vi "flat.vi"() -> ()   [LabVIEW 2020]
doc: "Recommended Input Signal: 100 kHz, 4 Vpp, sine wave\n\nDevices Supported: Refer to NI Example Finder\n\nThis example configures all the oscilloscope's vertical, horizontal, and triggering properties before every acquisition. It allows you to experiment with numerous configurations, including acquisition types and triggering modes, since it supports nearly the entire functionality of NI-SCOPE. However, it is may be more instructive to consult other examples about specific topics such as FlexRes, Random Interleaved Sampling, and Multi-Record to learn more about these features.\n\nMany parameters are included an the front panel of this example. Notice that the \"min sample rate\" is next to the \"actual sample rate,\" and similarly the \"min record length\" is near the \"actual record length.\" The \"min\" values are specified with the Configure Horizontal Timing VI. NI-SCOPE maintains a constant time per record for each acquisition. So when you specify a min sample rate and a min record length, this determines the amount of time the acquisition should take:\n\n time per record = min record length / min sampling rate. \n\nHowever, oscilloscopes support only a certain number of defined sampling rates, so if the value chosen is not a valid rate, it is rounded to the next higher rate, called the actual sample rate. The actual record length is then calculated in order to maintain the time per record. Both of these values are returned in this example so you can investigate the effects of parameter rounding with your oscilloscope. For more information about parameter coercions, see the NI High Speed Digitizers Help.\n\nThe enforce realtime property allows this example to use Random Interleaved Sampling. See the Random Interleaved Sampling example for more details.\n\nKeep in mind that not all digitizers/oscilloscopes support all the features in this example. The NI High Speed Digitizers Help includes a table of supported features for each device."
uses:
  <instrlib>/niFgen/niFgen.llb/niFgen Output Impedance.ctl
  <instrlib>/niDCPower/nidcpower.llb/niDCPower Source Mode.ctl
  <instrlib>/niDCPower/nidcpower.llb/niDCPower Output Function.ctl
  <instrlib>/niDCPower/nidcpower.llb/niDCPower Wait For Event - Event.ctl
  <instrlib>/niFgen/niFgen.llb/niFgen Output Mode.ctl
  <instrlib>/niFgen/niFgen.llb/niFgen Waveform Type.ctl
  <vilib>/measure/matone.llb/Extract Single Tone Information 1 Chan.vi
  <instrlib>/niScope/Acquire/Fetch/niScope Multi Fetch Cluster.vi
  <vilib>/measure/NI_MAPro.lvlib
panel:
  out "Vout":dbl[](array[numeric])
  out "Vin":dbl[](array[numeric])
  out "CH0 detected frequency":dbl format="%.2p"
  out "CH0 Spectrum(instantaneous)":cluster{"f0":dbl, "df":dbl, dbl[]}(graph)
  in  "Timeout (s)":dbl=5.0 format="%.2f"
  in  "% search":dbl=5.0
  in  "current level range":dbl=0.01 format="%#.6p"
  in  "voltage level range":dbl=10.0 format="%.6p"
  in  "Min record length":i32=1000000
  in  "Min Sample Rate (S/s)":dbl=5000000.0 format="%#_6p"
  in  "Load Current (A)":dbl=-0.01
  in  "Input Voltage (V)":dbl=7.5
  in  "SMU Load":refnum<k15>="SMU_Load"
  in  "SMU Source":refnum<k15>="SMU_Source"
  in  "Max Freq (Hz)":i32=1000000 format="%.0p"
  in  "Min Freq (Hz)":dbl(ring)=100.0 items=["10Hz"=10.0, "100Hz"=100.0, "1kHz"=1000.0, "100kHz"=100000.0]
  out "PSRR vs Frequency Graph":cluster{dbl, dbl}[](graph) caption="Input Voltage :\nLoad current :\nOutput voltage :"
  out "CH0":T1(graph)
  out "PSRR":dbl[](array[numeric])=[nan, nan, nan]
  in  "FGen Vpk-pk (V)":dbl=1.0 format="%#_2f"
  out "Current Freq(Hz)":dbl=300.0
  in  "FGEN Resource Name":refnum<k15>="FGEn"
  in  "Resource Name":refnum<k15>="PXI1Slot5" caption="Scope Resource Name"
  # "LDO_PSRR Measurement"
  # "Debug"
  # "Test Result"
  # "Configuration"
  # "SMU"
  # "Waveform Generator"
  # "Oscilloscope"
  # "Advance"
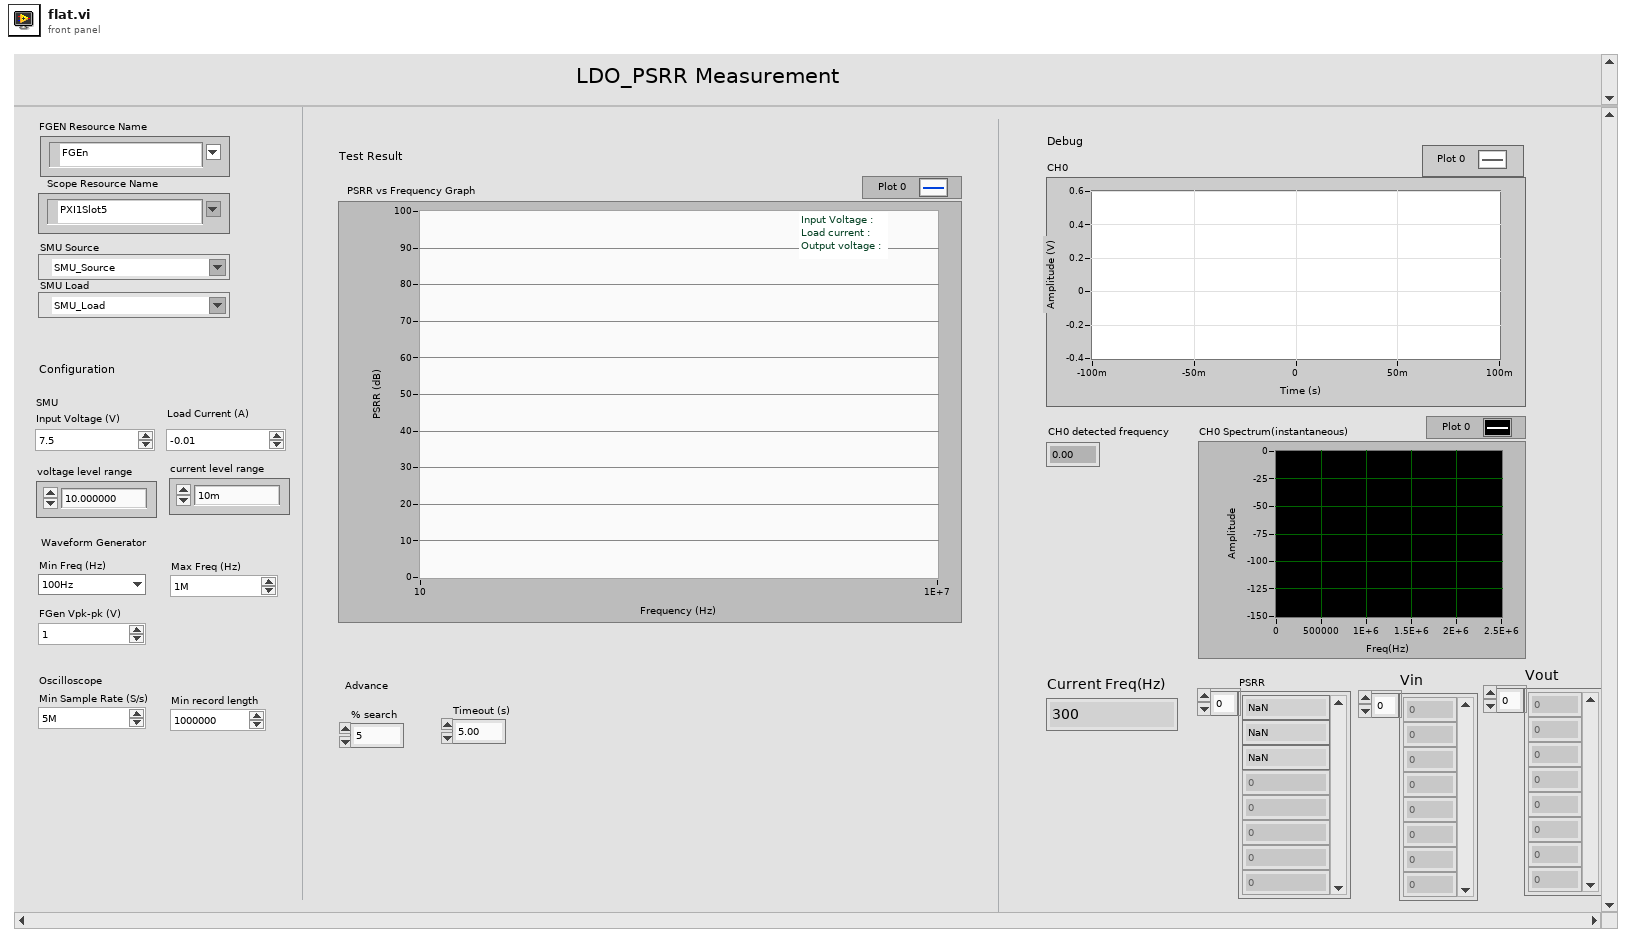
[diagram p1: front panel]
types:
  T1 = cluster{"relativeInitialX":dbl, "xIncrement":dbl, "wfm":dbl[]}
  T2 = typedef "niDCPower Output Function.ctl" = i32
  T3 = typedef "niDCPower Source Mode.ctl" = i32
  T4 = typedef "niDCPower Wait For Event - Event.ctl" = i32
  T5 = typedef "niFgen Output Impedance.ctl" = i32
  T6 = cluster{"approx freq. (optional)":dbl, "search (+/- % of Fsampl.)":dbl}
  T7 = enum32{"none", "input signal", "detected signal", "residual signal"}
  T8 = typedef "niFgen Waveform Type.ctl" = i32
  T9 = typedef "niFgen Output Mode.ctl" = u32
  T10 = cluster{"relativeInitialX":dbl, "xIncrement":dbl, "wfm":dbl[]}[]
  T11 = cluster{"exported time signal":waveform(dbl), "exported spectrum (dB)":cluster{"f0":dbl, "df":dbl, "dB Spectrum (Hann)":dbl[]}}
  T12 = cluster{"f0":dbl, "df":dbl, "dB Spectrum (Hann)":dbl[]}
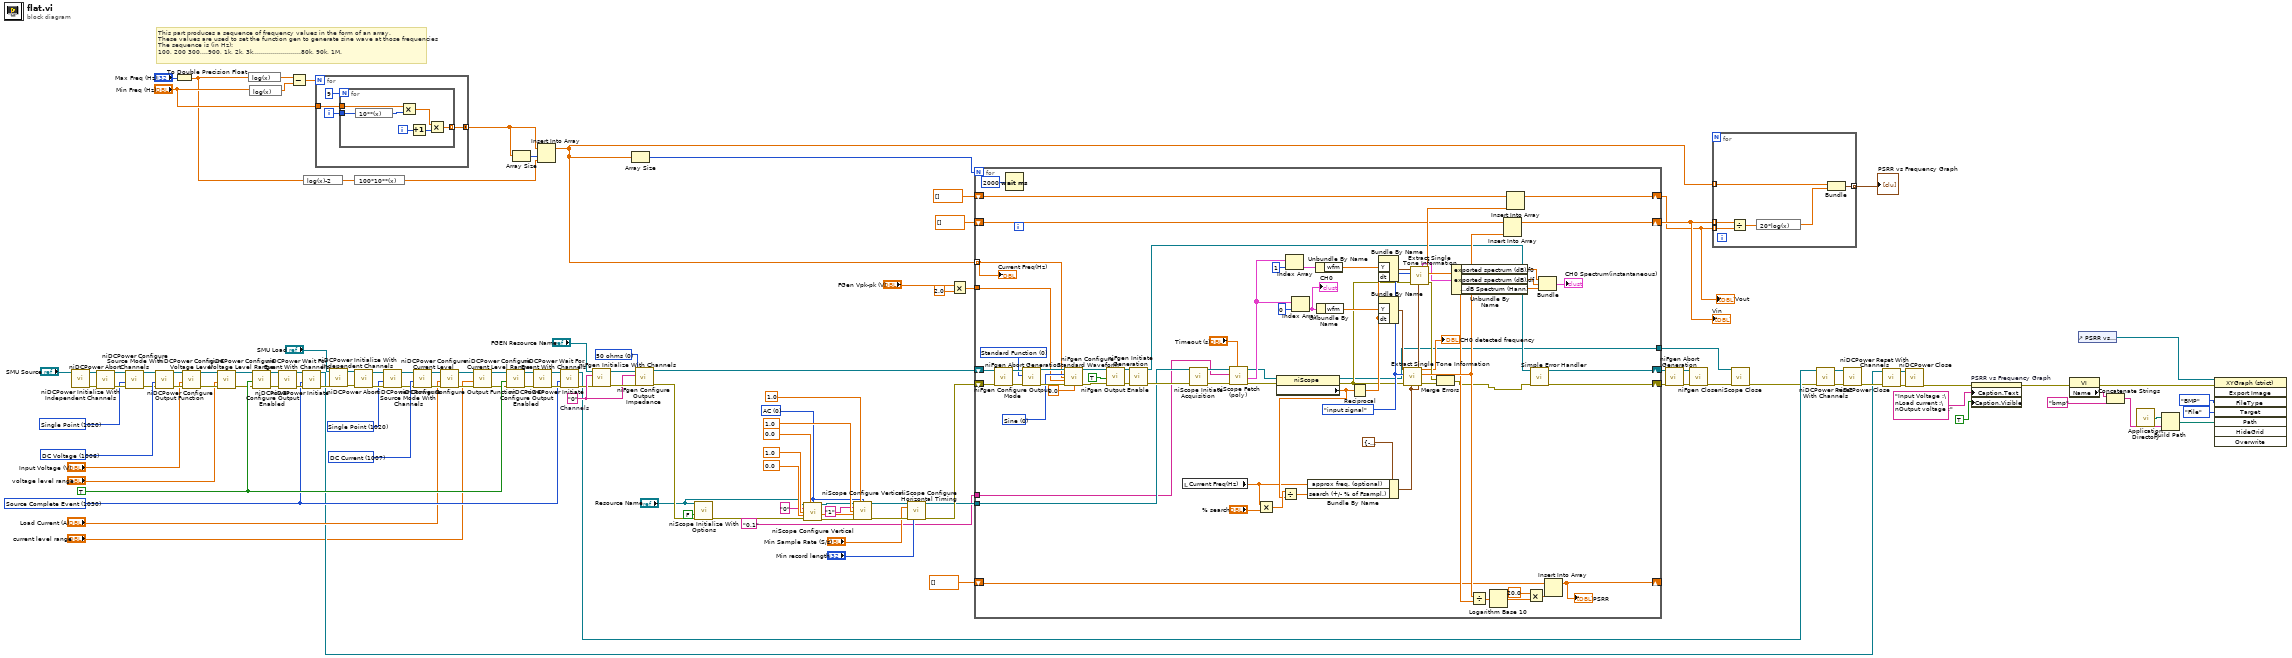
[diagram p0: block diagram]
diagram:
  w13 = 0 items=["AC", "DC", "Ground"] ("Vertical Coupling")
  w82 = T2 1007 items=["DC Voltage"=1006, "DC Current"=1007, "Pulse Voltage"=1049, "Pulse Current"=1050] ("output function")
  w79 = T3 1020 items=["Single Point"=1020, "Sequence"=1021] ("source mode")
  w66 = T4 1030 items=["Source Complete Event"=1030, "Measure Complete Event"=1031, "Sequence Iteration Complete Event"=1032, "Sequence Engine Done Event"=1033, "Pulse Complete Event"=1051, "Ready For Pulse Trigger Event"=1052] ("event")
  w67 = TRUE ("output enabled")
  w99 = T2 1006 items=["DC Voltage"=1006, "DC Current"=1007, "Pulse Voltage"=1049, "Pulse Current"=1050] ("output function")
  w96 = T3 1020 items=["Single Point"=1020, "Sequence"=1021] ("source mode")
  w108 = T5 0 items=["50 ohms", "75 ohms"] ("Impedance (default: 0=50 ohms)")
  w109 = "0"  # Channels
  # "This part produces a sequence of frequency values in the form of an array.\nThese values are used to set the function gen to generate sine wave at those frequencies\nThe sequence is (in Hz): \n100, 200 300,...900, 1k, 2k, 3k,.......................80k, 90k, 1M."
  n1 = call <instrlib>:"niDCPower Initialize With Independent Channels.vi"("resource name"="SMU Source") -> ("error out"=w87:errorcluster, "instrument handle out"=w86:refnum<k15>)  [unwired: 9 in]
  n2 = call <instrlib>:"niDCPower Abort.vi"("error in (no error)"=w87, "instrument handle"=w86) -> ("error out"=w100:errorcluster, "instrument handle out"=w101:refnum<k15>)  [unwired: 8 in]
  n3 = call <instrlib>:"niDCPower Configure Source Mode With Channels.vi"("error in (no error)"=w100, "source mode"=w96, "instrument handle"=w101) -> ("error out"=w98:errorcluster, "instrument handle out"=w97:refnum<k15>)  [unwired: 7 in]
  n4 = call <instrlib>:"niDCPower Configure Output Function.vi"("error in (no error)"=w98, "output function"=w99, "instrument handle"=w97) -> ("error out"=w95:errorcluster, "instrument handle out"=w94:refnum<k15>)  [unwired: 7 in]
  n5 = To Double Precision Float(number="Max Freq (Hz)") -> (double precision float=w46:dbl)
  n6 = call <instrlib>:"niDCPower Configure Voltage Level.vi"("error in (no error)"=w95, "voltage level"="Input Voltage (V)", "instrument handle"=w94) -> ("error out"=w93:errorcluster, "instrument handle out"=w44:refnum<k15>)  [unwired: 7 in]
  n7 = call <instrlib>:"niDCPower Configure Voltage Level Range.vi"("error in (no error)"=w93, "voltage level range"="voltage level range", "instrument handle"=w44) -> ("error out"=w45:errorcluster, "instrument handle out"=w43:refnum<k15>)  [unwired: 7 in]
  n8 = expression code="log(x)"(w46) -> (w53:dbl)
  n9 = expression code="log(x)"("Min Freq (Hz)") -> (w52:dbl)
  n10 = call <instrlib>:"niDCPower Configure Output Enabled.vi"("error in (no error)"=w45, "output enabled"=w67, "instrument handle"=w43) -> ("error out"=w92:errorcluster, "instrument handle out"=w91:refnum<k15>)  [unwired: 7 in]
  n11 = call <instrlib>:"niDCPower Initiate.vi"("error in (no error)"=w92, "instrument handle"=w91) -> ("error out"=w90:errorcluster, "instrument handle out"=w89:refnum<k15>)  [unwired: 8 in]
  n12 = Subtract(x=w53, y=w52) -> (x-y=w50:dbl)
  n13 = call <instrlib>:"niDCPower Wait For Event With Channels.vi"("error in (no error)"=w90, "event"=w66, "instrument handle"=w89) -> ("error out"=w69:errorcluster, "instrument handle out"=w58:refnum<k15>)  [unwired: 7 in]
  n14 = expression code="log(x)-2"(w46) -> (w51:dbl)
  n15 = for {
    N: w50 -> [_]
    tunnel: [w125] -> w55 mode=concatenating
    tunnel: "Min Freq (Hz)" -> [w122]
    i -> [w123]
    n16 = for {
      N: 9 -> [_]
      tunnel: w123 -> [w131]
      tunnel: [w130] -> w125 mode=indexing
      tunnel: w122 -> [w126]
      i -> [w132]
      n17 = expression code="10**(x)"(w131) -> (w127:i32)
      n18 = Multiply(x=w126, y=w127) -> (x*y=w128:dbl)
      n19 = Increment(x=w132) -> (x+1=w129:i32)
      n20 = Multiply(x=w128, y=w129) -> (x*y=w130:dbl)
    }
  }
  n21 = call <instrlib>:"niDCPower Initialize With Independent Channels.vi"("error in (no error)"=w69, "resource name"="SMU Load") -> ("error out"=w71:errorcluster, "instrument handle out"=w70:refnum<k15>)  [unwired: 8 in]
  n22 = expression code="100*10**(x)"(w51) -> (w56:dbl)
  n23 = call <instrlib>:"niDCPower Abort.vi"("error in (no error)"=w71, "instrument handle"=w70) -> ("error out"=w83:errorcluster, "instrument handle out"=w84:refnum<k15>)  [unwired: 8 in]
  n24 = call <instrlib>:"niDCPower Configure Source Mode With Channels.vi"("error in (no error)"=w83, "source mode"=w79, "instrument handle"=w84) -> ("error out"=w81:errorcluster, "instrument handle out"=w80:refnum<k15>)  [unwired: 7 in]
  n25 = call <instrlib>:"niDCPower Configure Output Function.vi"("error in (no error)"=w81, "output function"=w82, "instrument handle"=w80) -> ("error out"=w78:errorcluster, "instrument handle out"=w77:refnum<k15>)  [unwired: 7 in]
  n26 = call <instrlib>:"niDCPower Configure Current Level.vi"("error in (no error)"=w78, "current level"="Load Current (A)", "instrument handle"=w77) -> ("error out"=w72:errorcluster, "instrument handle out"=w40:refnum<k15>)  [unwired: 7 in]
  n27 = call <instrlib>:"niDCPower Configure Current Level Range.vi"("error in (no error)"=w72, "current level range"="current level range", "instrument handle"=w40) -> ("error out"=w41:errorcluster, "instrument handle out"=w39:refnum<k15>)  [unwired: 7 in]
  n28 = call <instrlib>:"niDCPower Configure Output Enabled.vi"("error in (no error)"=w41, "output enabled"=w67, "instrument handle"=w39) -> ("error out"=w76:errorcluster, "instrument handle out"=w75:refnum<k15>)  [unwired: 7 in]
  n29 = Array Size(array=w55) -> (size(s)=w54:i32)
  n30 = call <instrlib>:"niDCPower Initiate.vi"("error in (no error)"=w76, "instrument handle"=w75) -> ("error out"=w73:errorcluster, "instrument handle out"=w74:refnum<k15>)  [unwired: 8 in]
  n31 = Insert Into Array(array=w55, index=w54, new element=w56) -> (w47:dbl[])
  n32 = call <instrlib>:"niDCPower Wait For Event With Channels.vi"("error in (no error)"=w73, "event"=w66, "instrument handle"=w74) -> ("error out"=w68:errorcluster, "instrument handle out"=w57:refnum<k15>)  [unwired: 7 in]
  n33 = call <instrlib>:"niFgen Initialize With Channels.vi"("error in (no error)"=w68, "Channel Name"=w109, "Resource Name"="FGEN Resource Name") -> ("error out"=w110:errorcluster, "Instrument Handle Out"=w112:refnum<k15>)  [unwired: 7 in]
  n34 = Array Size(array=w47) -> (size(s)=w115:i32)
  n35 = call <instrlib>:"niFgen Configure Output Impedance.vi"("error in (no error)"=w110, "Impedance (default: 0=50 ohms)"=w108, "Channel Name"=w109, "Instrument Handle"=w112) -> ("error out"=w12:errorcluster, "Instrument Handle Out"=w111:refnum<k15>)  [unwired: 6 in]
  n36 = call <instrlib>:"niScope Initialize With Options.vi"("resource name"="Resource Name", "reset device"=FALSE ("Reset Device"), "error in"=w12) -> ("error out"=w23:errorcluster)  [unwired: 11 in, 1 out]
  n37 = call <instrlib>:"niScope Configure Vertical.vi"("instrument handle"="Resource Name", "vertical coupling"=w13, "channels"="0", "vertical range"=1.0 ("Vertical Range CH0"), "vertical offset"=0.0 ("Vertical Offset CH0"), "error in"=w23) -> ("instrument handle out"=w17:refnum<k15>, "error out"=w16:errorcluster)  [unwired: 8 in]
  n38 = call <instrlib>:"niScope Configure Vertical.vi"("instrument handle"=w17, "probe attenuation"=1.0 ("Probe Attenuation"), "vertical coupling"=w13, "channels"="1", "vertical range"=1.0 ("Vertical Range CH1"), "vertical offset"=0.0 ("Vertical Offset CH1"), "error in"=w16) -> ("instrument handle out"=w6:refnum<k15>, "error out"=w8:errorcluster)  [unwired: 7 in]
  n39 = call <instrlib>:"niScope Configure Horizontal Timing.vi"("instrument handle"=w6, "min sample rate"="Min Sample Rate (S/s)", "error in"=w8, "min record length"="Min record length") -> ("instrument handle out"=w5:refnum<k15>, "error out"=w7:errorcluster)  [unwired: 10 in]
  n40 = Multiply(x="FGen Vpk-pk (V)", y=2.0) -> (x*y=w117:dbl)
  n41 = for {
    N: w115 -> [_]
    shift-right: [w184] -> w119
    shift-left: w111 -> [w186]
    shift-right: [w183] -> w118
    shift-left: w7 -> [w185]
    tunnel: w47 -> [w172] mode=indexing
    tunnel: w117 -> [w181]
    shift-right: [w170] -> _
    shift-left: dbl[] [] -> [w171]
    shift-right: [w174] -> w102
    shift-left: dbl[] [] -> [w176]
    shift-right: [w173] -> w103
    shift-left: dbl[] [] -> [w175]
    tunnel: w5 -> [w134]
    tunnel: "0,1" ("Channel Name") -> [w133]
    tunnel: [w136] -> w11
    w157 = T7."input signal" ("export mode")
    w188 = T8 0 items=["Sine", "Square", "Triangle", "Ramp Up", "Ramp Down", "DC", "Noise", "User"] ("Waveform")
    w193 = T9 0 items=["Standard Function", "Frequency List", "Arbitrary Waveform", "Arbitrary Sequence", "Script"] ("output mode")
    n42 = call <instrlib>:"niFgen Abort Generation.vi"("error in (no error)"=w185, "Instrument Handle"=w186) -> ("error out"=w195:errorcluster, "Instrument Handle Out"=w196:refnum<k15>)  [unwired: 8 in]
    n43 = Wait (ms)(milliseconds to wait=u32 2000) -> ()  [unwired: 1 out]
    n44 = call <instrlib>:"niFgen Configure Output Mode.vi"("error in (no error)"=w195, "Output Mode (default: 0=Standard Function)"=w193, "Instrument Handle"=w196) -> ("error out"=w190:errorcluster, "Instrument Handle Out"=w189:refnum<k15>)  [unwired: 6 in]
    n45 = call <instrlib>:"niFgen Configure Standard Waveform.vi"("Instrument Handle"=w189, "Waveform"=w188, "Frequency"=w172, "Amplitude"=w181, "error in (no error)"=w190, "DC Offset"=0.0) -> ("Instrument Handle Out"=w192:refnum<k15>, "error out"=w191:errorcluster)  [unwired: 8 in]
    n46 = call <instrlib>:"niFgen Output Enable.vi"("error in (no error)"=w191, "Output Enable (default: True)"=TRUE ("output enable"), "Instrument Handle"=w192) -> ("error out"=w197:errorcluster, "Instrument Handle Out"=w198:refnum<k15>)  [unwired: 7 in]
    n47 = call <instrlib>:"niFgen Initiate Generation.vi"("error in (no error)"=w197, "Instrument Handle"=w198) -> ("error out"=w135:errorcluster, "Instrument Handle Out"=w184:refnum<k15>)  [unwired: 8 in]
    n48 = local read "Current Freq(Hz)"() -> (w147:dbl)
    n49 = call <instrlib>:"niScope Initiate Acquisition.vi"("instrument handle"=w134, "error in"=w135) -> ("instrument handle out"=w168:refnum<k15>, "error out"=w167:errorcluster)  [unwired: 12 in]
    n50 = call-poly <instrlib>:"niScope Fetch (poly).vi"("timeout"="Timeout (s)", "error in"=w167, "channels"=w133, "instrument handle"=w168) -> ("error out"=w161:errorcluster, "waveform"=w166:T10, "instrument handle out"=w162:refnum<k15>)  [unwired: 4 in, 1 out]
    n51 = Multiply(x=w147, y="% search") -> (x*y=w149:dbl)
    n52 = property class="niScope"(reference=w162, error in=w161) -> (reference out=w136:refnum<k15>, error out=w154:errorcluster, "Horizontal:Actual Sample Rate"=w148:dbl)
    n53 = Divide(x=w149, y=w148) -> (x/y=w145:dbl)
    n54 = Index Array(array=w166, index=1) -> (element=w151:T1)
    n55 = Index Array(array=w166, index=0) -> (element=w150:T1)
    "CH0" <- w150
    n56 = Bundle By Name(cluster=T6 {"approx freq. (optional)"=-1.0, "search (+/- % of Fsampl.)"=5.0} ("Set Frequency(Hz)"), "approx freq. (optional)"=w147, "search (+/- % of Fsampl.)"=w145) -> (w159:T6)
    n57 = Unbundle By Name(w151) -> ("wfm"=w156:dbl[])
    n58 = Unbundle By Name(w150) -> ("wfm"=w155:dbl[])
    n59 = Reciprocal(x=w148) -> (1/x=w163:dbl)
    n60 = Bundle By Name("Y"=w156, "dt"=w163) -> (w138:waveform(dbl))  [unwired: 1 in]
    n61 = Bundle By Name("Y"=w155, "dt"=w163) -> (w160:waveform(dbl))  [unwired: 1 in]
    n62 = call-poly <vilib>:"Extract Single Tone Information.vi"("advanced search"=w159, "error in (no error)"=w154, "export mode"=w157, "time signal in"=w160) -> ("error out"=w153:errorcluster, "detected amplitude"=w200:dbl, "detected frequency"=→"CH0 detected frequency":dbl)  [unwired: 2 in, 3 out]
    n63 = call-poly <vilib>:"Extract Single Tone Information.vi"("advanced search"=w159, "error in (no error)"=w154, "export mode"=w157, "time signal in"=w138) -> ("error out"=w152:errorcluster, "detected amplitude"=w199:dbl, "exported signals"=w140:T11)  [unwired: 2 in, 3 out]
    n64 = Merge Errors(w152, w153) -> (w137:errorcluster)
    n65 = Unbundle By Name(w140) -> ("exported spectrum (dB).f0"=w144:dbl, "exported spectrum (dB).df"=w141:dbl, "exported spectrum (dB).dB Spectrum (Hann)"=w143:dbl[])
    n66 = Divide(x=w200, y=w199) -> (x/y=w178:dbl)
    n67 = Logarithm Base 10(1:w178) -> (0:w179:dbl)
    n68 = Insert Into Array(array=w175, new element=w200) -> (w173:dbl[])  [unwired: 1 in]
    n69 = Insert Into Array(array=w176, new element=w199) -> (w174:dbl[])  [unwired: 1 in]
    n70 = Multiply(x=20.0, y=w179) -> (x*y=w177:dbl)
    n71 = call <vilib>:"Simple Error Handler.vi"("error in (no error)"=w137) -> ("error out"=w183:errorcluster)  [unwired: 4 in, 4 out]
    n72 = Bundle("f0"=w144, "df"=w141, "dB Spectrum (Hann)"=w143) -> (→"CH0 Spectrum(instantaneous)":T12)  [unwired: 1 in]
    n73 = Insert Into Array(array=w171, new element=w177) -> (w170:dbl[])  [unwired: 1 in]
    "PSRR" <- w170
    "Current Freq(Hz)" <- w172
  }
  "Vin" <- w103
  "Vout" <- w102
  n74 = call <instrlib>:"niFgen Abort Generation.vi"("error in (no error)"=w118, "Instrument Handle"=w119) -> ("error out"=w120:errorcluster, "Instrument Handle Out"=w121:refnum<k15>)  [unwired: 8 in]
  n75 = call <instrlib>:"niFgen Close.vi"("error in (no error)"=w120, "Instrument Handle"=w121) -> ("error out"=w10:errorcluster)  [unwired: 9 in]
  n76 = for {
    tunnel: w103 -> [w206] mode=indexing
    tunnel: w102 -> [w205] mode=indexing
    tunnel: w47 -> [w202] mode=indexing
    tunnel: [w203] -> w104 mode=indexing
    n77 = Divide(x=w206, y=w205) -> (x/y=w204:dbl)
    n78 = expression code="20*log(x)"(w204) -> (w201:dbl)
    n79 = Bundle(w202, w201) -> (w203:cluster{dbl, dbl})  [unwired: 1 in]
  }
  "PSRR vs Frequency Graph" <- w104
  n80 = call <instrlib>:"niScope Close.vi"("instrument handle"=w11, "error in"=w10) -> ("error out"=w9:errorcluster)  [unwired: 13 in]
  n81 = call <instrlib>:"niDCPower Reset With Channels.vi"("error in (no error)"=w9, "instrument handle"=w57) -> ("error out"=w63:errorcluster, "instrument handle out"=w62:refnum<k15>)  [unwired: 8 in]
  n82 = call <instrlib>:"niDCPower Close.vi"("error in (no error)"=w63, "instrument handle"=w62) -> ("error out"=w59:errorcluster)  [unwired: 9 in]
  n83 = call <instrlib>:"niDCPower Reset With Channels.vi"("error in (no error)"=w59, "instrument handle"=w58) -> ("error out"=w60:errorcluster, "instrument handle out"=w61:refnum<k15>)  [unwired: 8 in]
  n84 = call <instrlib>:"niDCPower Close.vi"("error in (no error)"=w60, "instrument handle"=w61) -> ("error out"=w37:errorcluster)  [unwired: 9 in]
  n85 = property on="PSRR vs Frequency Graph" class="XYGraph (strict)"(error in=w37, "Caption.Text"="Input Voltage :\nLoad current :\nOutput voltage :", "Caption.Visible"=TRUE) -> (error out=w27:errorcluster)  [unwired: 1 in, 1 out]
  n86 = property class="VI"(error in=w27) -> (error out=w33:errorcluster, "Name"=w32:string)  [unwired: 1 in, 1 out]
  n87 = control-ref of="PSRR vs Frequency Graph"() -> (w36:refnum<vi>)
  n88 = Concatenate Strings(w32, "bmp" ("string")) -> (w29:string)
  n89 = call <vilib>:"Application Directory.vi"() -> ("Application Directory"=w30:path)
  n90 = Build Path(base path=w30, name or relative path=w29) -> (appended path=w28:path)
  n91 = invoke class="XYGraph (strict)" method="Export Image"(reference=w36, error in=w33, "FileType"=enum32{"BMP", "EPS", "EMF", "PICT"}."BMP" ("File Type"), "Target"=enum32{"File", "Clipboard"}."File", "Path"=w28) -> ()  [unwired: 3 in, 8 out]
